vi "Unmarshal.vi"(8 "error in (no error)":errorcluster, 10 "Buffer":u8[](array[numeric]), 11 "int32 in":refnum<class "uint32.lvclass">) -> (0 "error out":errorcluster, 2 "Buffer Count":i32=8, 3 "int32 out":refnum<class "uint32.lvclass">)   [LabVIEW 2020, in "Protobuf RAW.lvlib" / "uint32.lvclass"]
uses:
  uint32.lvclass
  uint32.lvclass/uint32.ctl
  Protobuf RAW.lvlib
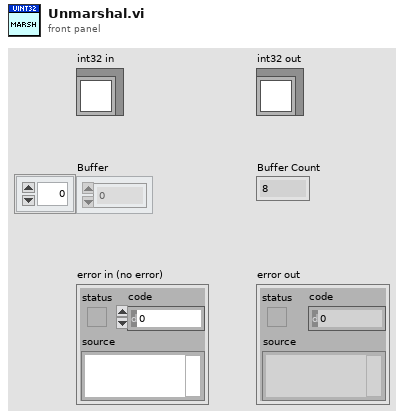
[diagram p1: front panel]
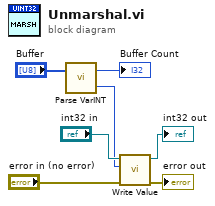
[diagram p0: block diagram]
diagram:
  n1 = call "Parse VarINT.vi"("Buffer"="Buffer") -> ("Numeric"=w1:u64, "Bytes"=→"Buffer Count":i32)  [unwired: 1 in]
  n2 = call "Write Value.vi"("error in (no error)"="error in (no error)", "Value"=w1, "int32 in"="int32 in") -> ("error out"=→"error out":errorcluster, "int32 out"=→"int32 out":refnum<class "uint32.lvclass">)  [unwired: 7 in]
